vi "CreateTxSession.vi"(8 "error in (no error)":errorcluster, 11 "NI-XNET in":refnum<class "NI-XNET.lvclass">) -> (0 "error out":errorcluster, 3 "NI-XNET out":refnum<class "NI-XNET.lvclass">)   [LabVIEW 2023, in "HardwareAbstractionLayer_LVOOP.lvlib" / "CAN HAL Lib.lvlib" / "NI-XNET.lvclass"]
uses:
  NI-XNET.lvclass
  NI-XNET.lvclass/NI-XNET.ctl
  <vilib>/xnet/xnet.llb/XNET Create Session (Frame Output Stream).vi
  <resource>/objmgr/xnet.rc
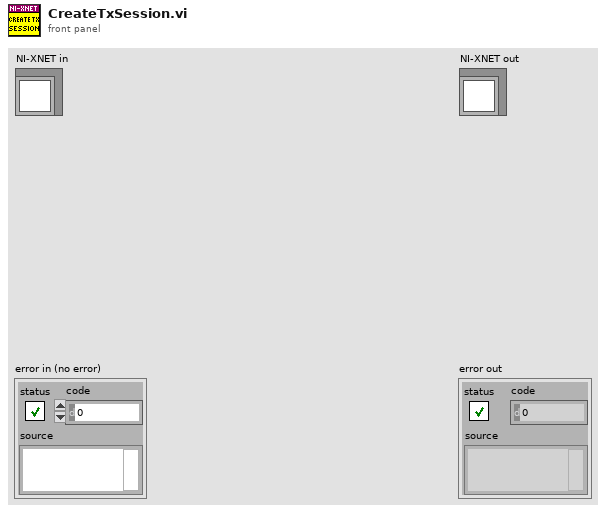
[diagram p1: front panel]
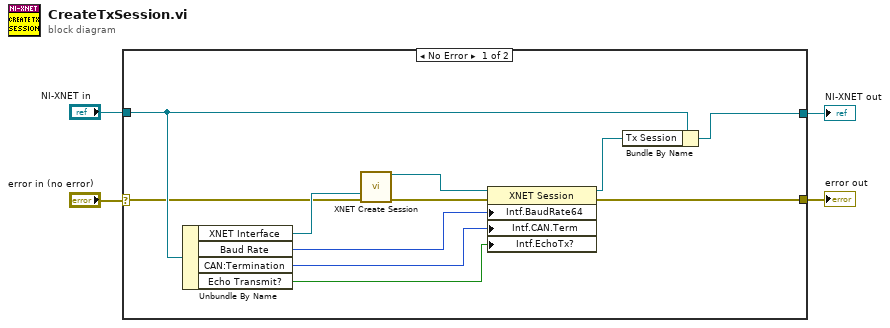
[diagram p0: block diagram]
diagram:
  n1 = case shown="No Error" "error in (no error)" {
    selector: "error in (no error)" -> [w6 w16]
    tunnel: "NI-XNET in" -> [w10 w17]
    tunnel: [w8 w17] -> w3
    tunnel: [w7 w16] -> w1
    frame No Error {
      n2 = Unbundle By Name(w10) -> ("XNET Interface"=w13:refnum<k21>, "Baud Rate"=w12:u64, "CAN:Termination"=w11:u32, "Echo Transmit?"=w5:bool)
      n3 = call-poly <vilib>:"XNET Create Session.vi"("interface"=w13, "error in (no error)"=w6) -> ("session out"=w15:refnum<k21>, "error out"=w14:errorcluster)  [unwired: 12 in]
      n4 = property class="XNET Session"(reference=w15, error in=w14, "Intf.BaudRate64"=w12, "Intf.CAN.Term"=w11, "Intf.EchoTx?"=w5) -> (reference out=w9:refnum<k21>, error out=w7:errorcluster)
      n5 = Bundle By Name(cluster=w10, "Tx Session"=w9) -> (w8:refnum<class "NI-XNET.lvclass">)
    }
    frame Error {
    }
  }
  "error out" <- w1
  "NI-XNET out" <- w3
